vi "LWXPS_XYLineArcVerification.vi"(6 "LabVIEW error IN":errorcluster, 7 "Trajectory file name":string, 8 "XY group name":string, 9 "XPS Reference IN":refnum<k24>) -> (0 "LabVIEW error OUT":errorcluster, 1 "XPS Error String":string, 2 "Returned error code":i32, 3 "XPS Reference OUT":refnum<k24>)   [LabVIEW 2014]
uses:
  D:/XPSQ8_LabView_Library/Development/Source/Dll/Newport.XPS.CommandInterface.dll
  Dll/Newport.XPS.CommandInterface.dll
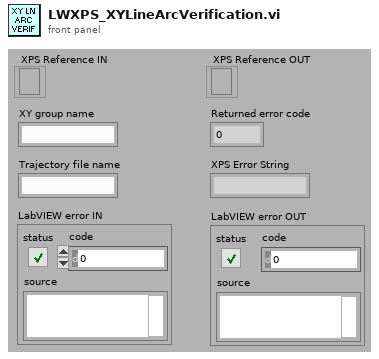
[diagram p1: front panel]
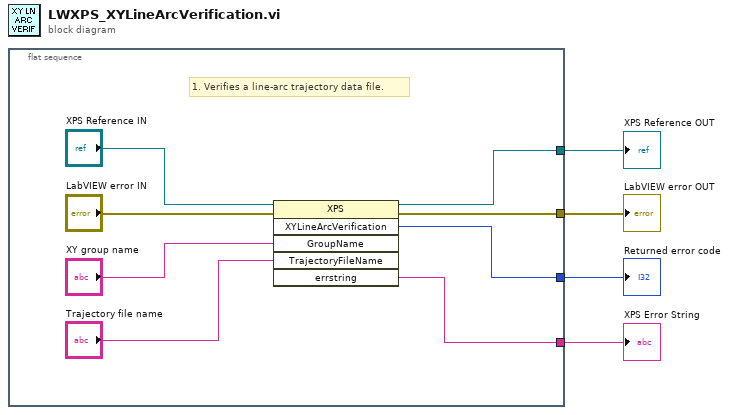
[diagram p0: block diagram]
diagram:
  n1 = flat-sequence {
    tunnel: [w10] -> w4
    tunnel: [w9] -> w3
    tunnel: [w11] -> w2
    tunnel: [w7] -> w1
    frame #0 {
      # "1. Verifies a line-arc trajectory data file."
      n2 = invoke class="XPS" method="XYLineArcVerification"(reference="XPS Reference IN", error in="LabVIEW error IN", "GroupName"="XY group name", "TrajectoryFileName"="Trajectory file name") -> (reference out=w10:refnum<k24>, error out=w9:errorcluster, "XYLineArcVerification"=w11:i32, "errstring"=w7:string)  [unwired: 2 in, 2 out]
    }
  }
  "XPS Error String" <- w1
  "XPS Reference OUT" <- w4
  "LabVIEW error OUT" <- w3
  "Returned error code" <- w2
